vi "Field_C.vi"(8 "Queue to master":T10, 11 "Module queue":T10) -> ()   [LabVIEW 2024, in "Magnet module.lvlib"]
doc: "Magnet module controls: power supply unit (PSU/SMS) and temperature monitor (TM/LSC218).\nPSU controls mainly: switch heater and ramping of current which runs throught coil.\nTM controls temperature of switch, coil and cryostat.\nMessage for magnet is a cluster that contains: {(enum) Command , (variant) Data}\nFor simplifieing of documentation, the Command is noted as a name of instruction, and Data is represented by a requered datatype (mostly cluster) name.\nCommands:\nInitialize(Magnet Config Constants) - Sugesstion: Load configuration constants from configuration file.\nSet field (Set field{B, R, cr}) - B-field[T], R-ramp[A/s], cr - custom ramp[bool].\nSwitch mode(mode) - to persistant, or to ramping.\nBlackout() - undone functionality of emergency deenergizing.\nUpdate() - Important! This triggers update of data from instruments. Shoud occure in regular intervals as priority message.\nResponses:\nMagnet initialized ();\nTM revision(temperature monitor revision);\nMagnet init error(error);\nSetting field(Set Field{B, R, cr});\nWarning(string);\nSwitching to(mode);\nUpdate error(error);\nTM update(TM sensors);\nPSU update(PSU data);\nMagnet status();"
uses:
  Magnet module.lvlib
  ctl/SetField data.ctl
  ctl/RampingOutput.ctl
  ctl/Magnet mode.ctl
  ctl/Overall status.ctl
  ctl/Magnet config constants.ctl
  ctl/Cryostat temperature sensors.ctl
  Messenger service/Data types/Module name.ctl
  <instrlib>/SMS drivers/Public/PSU Status.ctl
  <instrlib>/SMS drivers/Cryogenic Ltd SMSXXX.lvlib
  ctl/Magnet Orders.ctl
  ctl/MSG to magnet.ctl
  ctl/Magnet mode public.ctl
  ctl/Actual magnet state.ctl
  Messenger service/Data types/Mailbox address.ctl
  Messenger service/MessengerLib.lvlib
panel:
  out "Time stamp":dbl format="%<%H:%M:%S%3u\n%Y/%m/%d>T"
  out "Connected":bool
  out "Magnet Constants":T1={"Switch resistant [K]"=5.0, "Switch superconducting [K]"=4.0, "First stage critical temperature [K]"=50.0, "Second stage critical temperature [K]"=5.0, "Inner magnet critical temperature [K]"=6.0, "Outer magnet critical temperature [K]"=5.0, "Field Constant [T/A]"=0.14911, "Maximum Current [A]"=107.3, "Maximum field [T]"=16.0, "Maximum source ramp [A/s]"=0.5, "Source precision [T]"=2e-05, "Ramp limits [A/s]"=[0.0506, 0.038, 0.0285, 0.0213, 0.0104], "Field limits [T]"=[3.0, 9.6, 13.3, 15.5, 16.0], "SMS"="", "LSC218"=""}
  out "Overall status":T2={"Desired"={"Field [T]"=0.0, "Ramp [T/s]"=0.0, "Custom Ramp?"=TRUE, "Mode"=enum."Persistant"}, "Actual"={"Mode"=enum."Persistant", "Ramping output"=enum."At Target", "Ready for change"=FALSE, "Switch heater"=FALSE, "Cooler Overheat"=FALSE, "Coil overheat"=FALSE, "Energized"=FALSE, "Output [T]"=0.0, "Field [T]"=0.0, "Ramp[T/s]"=0.0, "Switch\ntemperature [K]"=1.0, "Voltage [V]"=0.0, "Current direction"=FALSE}}
  out "Temperatures":T8 {"Time stamp" format="%<%H:%M:%S%2u\n%Y/%m/%d>T"}
  out "PSU Status Out":T9 {"Trip Current" format="%.3f"; "Trip Field" format="%.4f"; "Voltage" format="%.2f"; "Field Constant" format="%.6f"; "MID Setpoint (T)" format="%.4f"; "MID Setpoint (A)" format="%.3f"; "MAX Setpoint (T)" format="%.4f"; "MAX Setpoint (A)" format="%.3f"; "Heater Voltage" format="%.2f"; "V Limit (V)" format="%.2f"; "Ramp Rate (A/s)" format="%.3f"; "Output (A)" format="%.3f"; "Output (T)" format="%.4f"; "Persistent Current" format="%.3f"; "Persistent Field" format="%.4f"}
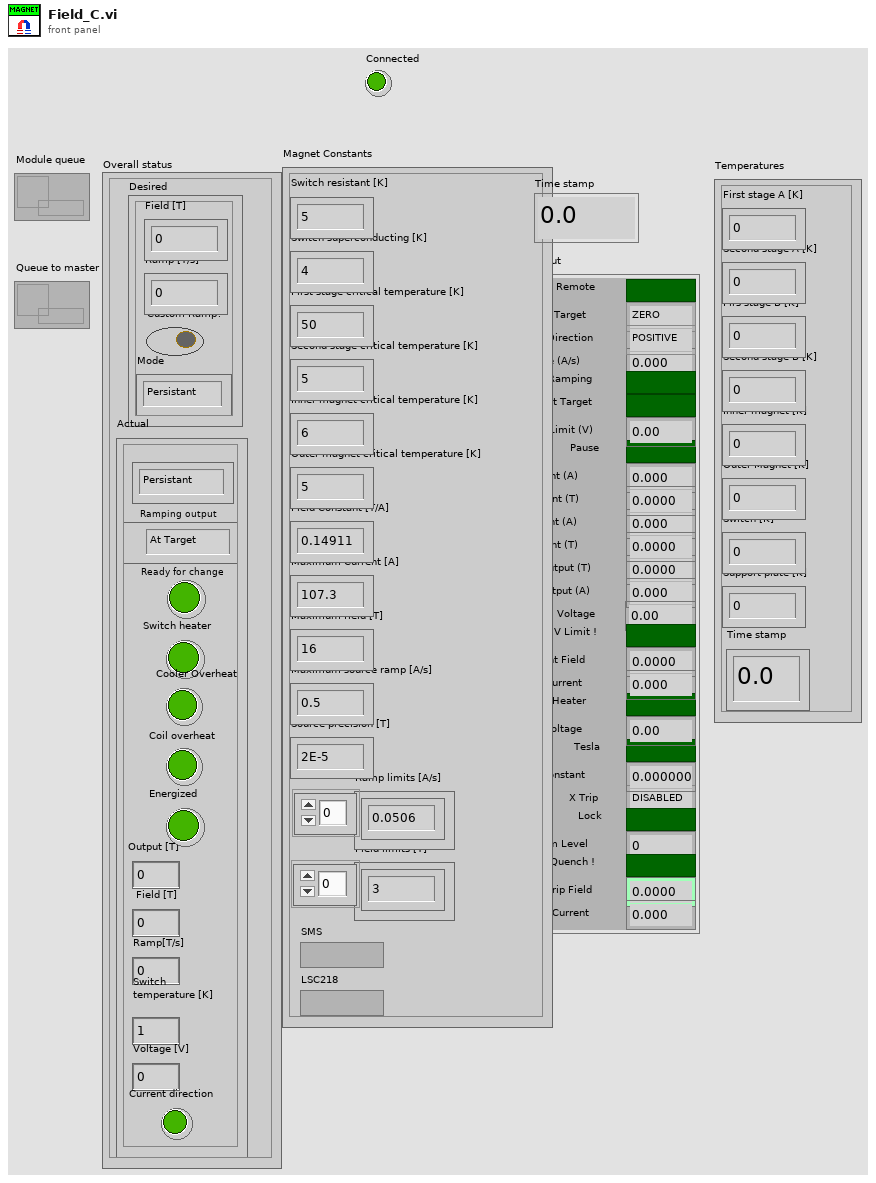
[diagram p1: front panel]
types:
  T1 = typedef "Magnet module.lvlib/Magnet config constants.ctl" = cluster{"Switch resistant [K]":dbl, "Switch superconducting [K]":dbl, "First stage critical temperature [K]":dbl, "Second stage critical temperature [K]":dbl, "Inner magnet critical temperature [K]":dbl, "Outer magnet critical temperature [K]":dbl, "Field Constant [T/A]":dbl, "Maximum Current [A]":dbl, "Maximum field [T]":dbl, "Maximum source ramp [A/s]":dbl, "Source precision [T]":dbl, "Ramp limits [A/s]":dbl[], "Field limits [T]":dbl[], "SMS":refnum<visa-resource-name>, "LSC218":refnum<visa-resource-name>}
  T2 = typedef "Magnet module.lvlib/Overall status.ctl" = cluster{"Desired":T3, "Actual":T5}
  T3 = typedef "Magnet module.lvlib/SetField data.ctl" = cluster{"Field [T]":dbl, "Ramp [T/s]":dbl, "Custom Ramp?":bool, "Mode":T4}
  T4 = typedef "Magnet module.lvlib/Magnet mode public.ctl" = enum16{"Persistant", "Ramping"}
  T5 = typedef "Magnet module.lvlib/Actual magnet state.ctl" = cluster{"Mode":T6, "Ramping output":T7, "Ready for change":bool, "Switch heater":bool, "Cooler Overheat":bool, "Coil overheat":bool, "Energized":bool, "Output [T]":dbl, "Field [T]":dbl, "Ramp[T/s]":dbl, "Switch\ntemperature [K]":dbl, "Voltage [V]":dbl, "Current direction":bool}
  T6 = typedef "Magnet module.lvlib/Magnet mode.ctl" = enum16{"Persistant", "Switching", "Ramping", "Quenched"}
  T7 = typedef "Magnet module.lvlib/RampingOutput.ctl" = enum16{"At Target", "Go up", "Go down"}
  T8 = typedef "Magnet module.lvlib/Cryostat temperature sensors.ctl" = cluster{"First stage A [K]":dbl, "Second stage A [K]":dbl, "Firs stage B [K]":dbl, "Second stage B [K]":dbl, "Inner magnet [K]":dbl, "Outer Magnet [K]":dbl, "Switch [K]":dbl, "Support plate [K]":dbl, "Time stamp":dbl}
  T9 = typedef "Cryogenic Ltd SMSXXX.lvlib/PSU Status.ctl" = cluster{"Ramp Target":enum16{"ZERO", "MID", "MAX"}, "Pause":bool, "Switch Heater":bool, "Persistent Field":dbl, "Persistent Current":dbl, "Tesla":bool, "Output (T)":dbl, "Output (A)":dbl, "X Trip":enum16{"DISABLED", "ENABLED", "ACTIVE"}, "Ramp Rate (A/s)":dbl, "V Limit (V)":dbl, "Heater Voltage":dbl, "MAX Setpoint (A)":dbl, "MAX Setpoint (T)":dbl, "MID Setpoint (A)":dbl, "MID Setpoint (T)":dbl, "Lock":bool, "Field Constant":dbl, "Remote":bool, "Direction":enum16{"POSITIVE", "NEGATIVE", "OPEN", "UNIPOLAR"}, "Helium Level":u16, "Quench !":bool, "Voltage":dbl, "V Limit !":bool, "Ramping":bool, "At Target":bool, "Trip Field":dbl, "Trip Current":dbl}
  T10 = typedef "MessengerLib.lvlib/Mailbox address.ctl" = refnum<queue>
  T11 = enum16{"Begin", "Idle", "Connect", "UpdateAll", "UpdateQuick", "Set field", "Set mode", "Emergency", "Disconnect", "Exit"}
  T12 = typedef "Module name.ctl" = enum16{"Emty", "Magnet", "VTI", "Excitation", "Servo", "Acquisition", "Rotator", "Digitizer", "SMU2450", "Carousel", "Multimeter", "Tmp monitor", "Power monitor"}
  T13 = typedef "Magnet module.lvlib/Magnet Orders.ctl" = enum16{"Ignore", "Connect", "Update", "Switch mode", "Set field", "Stop ramping", "Equalize output", "Zero output", "Flip polarity", "Blackout", "Set timer", "Eval temperatures", "Disconnect"}
  T14 = typedef "Magnet module.lvlib/MSG to magnet.ctl" = cluster{"Order":T13, "Data":variant}
  T15 = enum16{"POSITIVE", "NEGATIVE", "OPEN", "UNIPOLAR"}
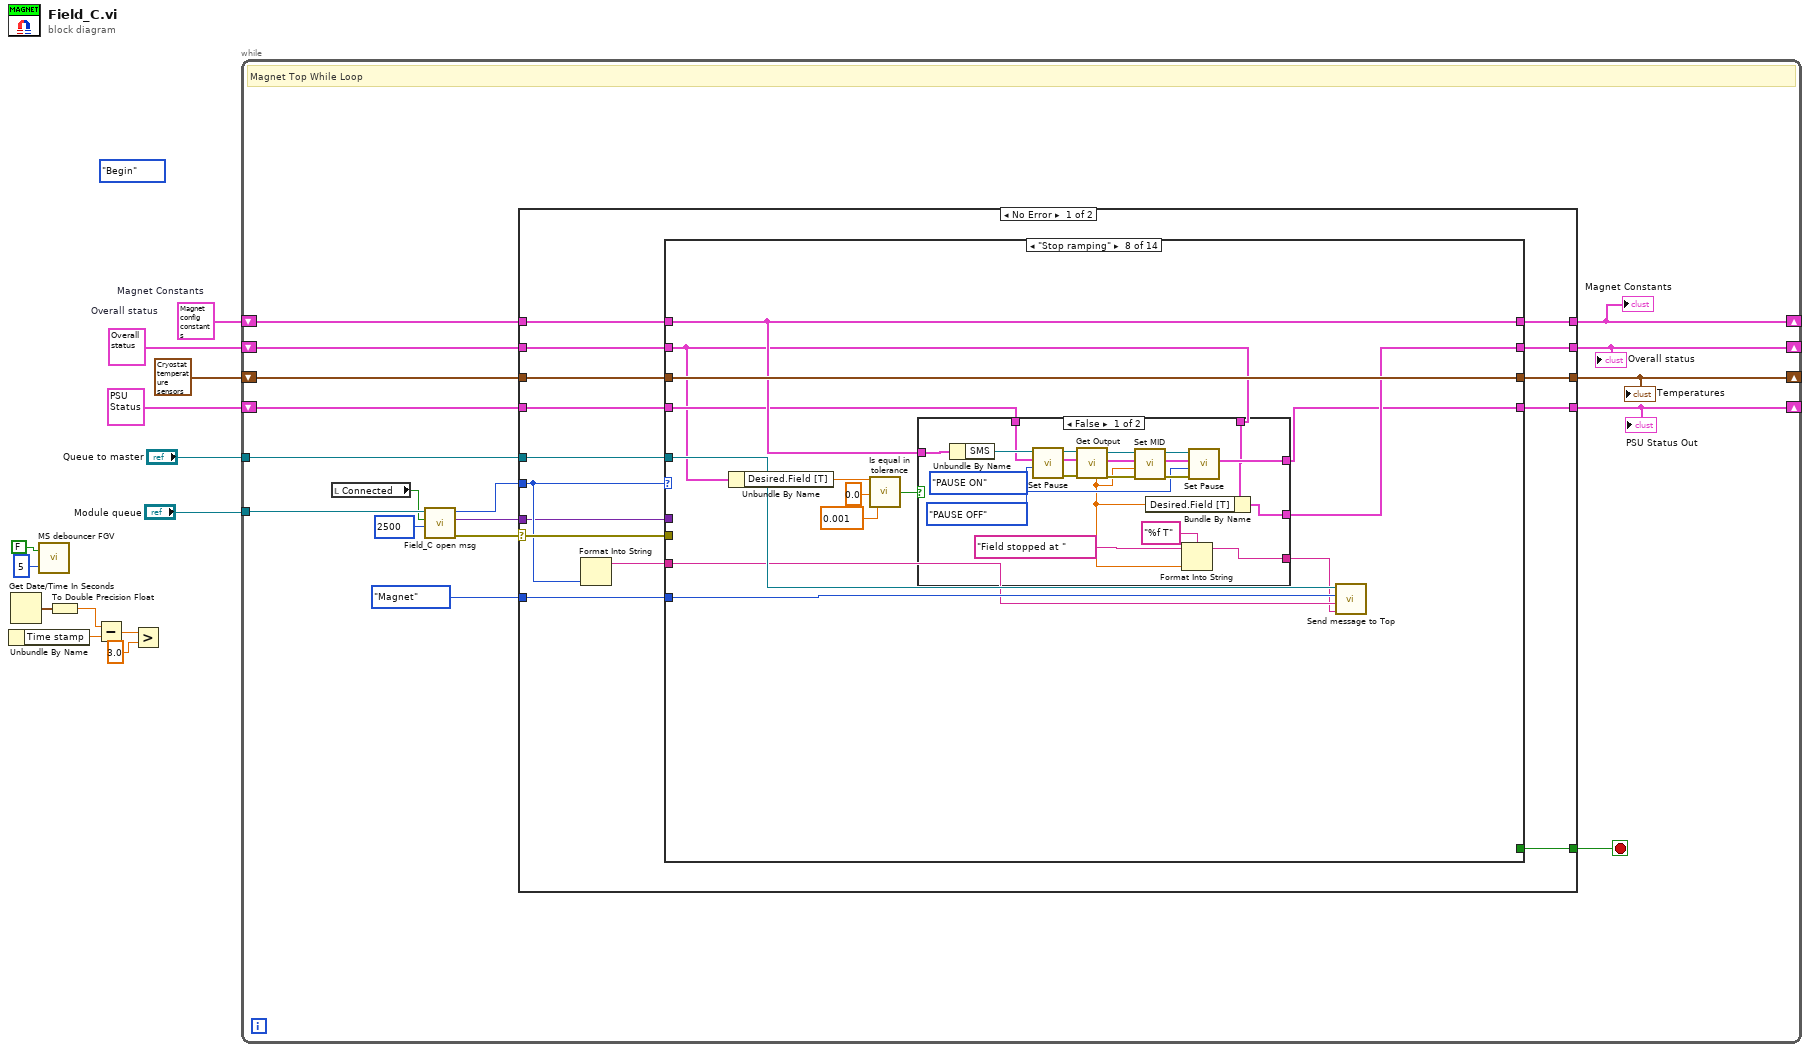
[diagram p0: block diagram]
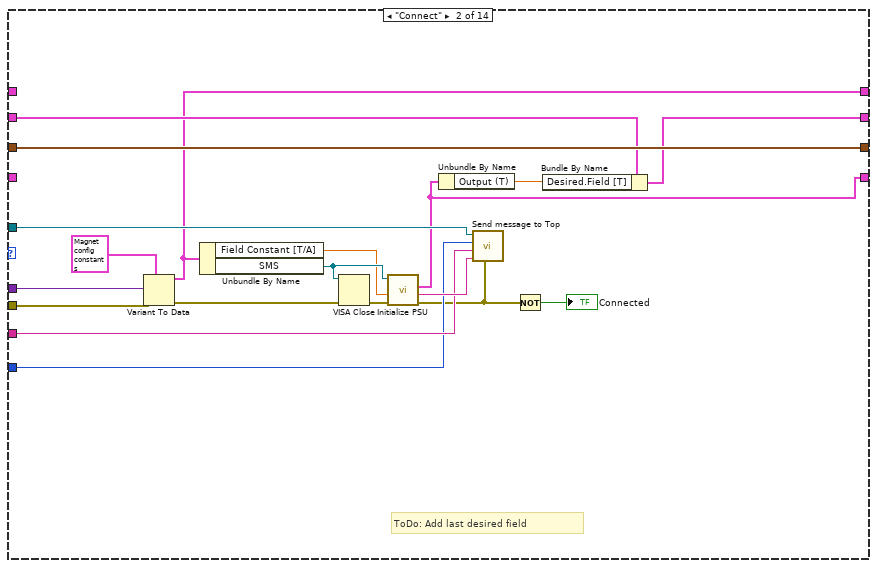
[diagram p3: hidden frame]
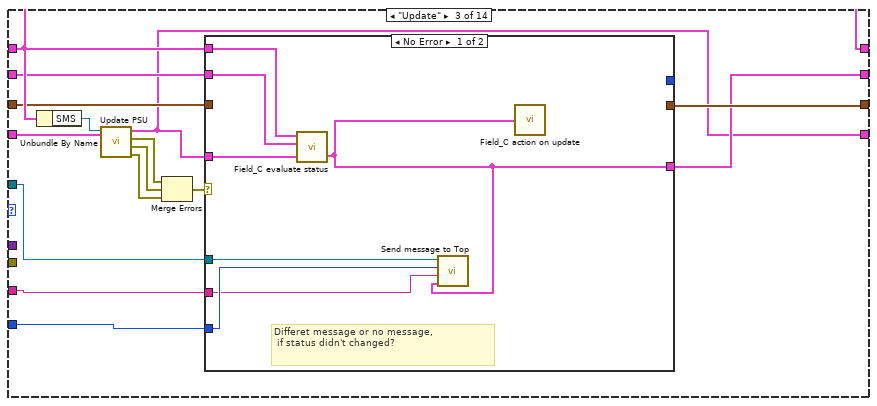
[diagram p4: hidden frame]
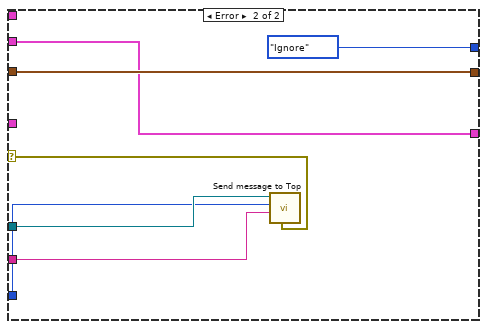
[diagram p5: hidden frame]
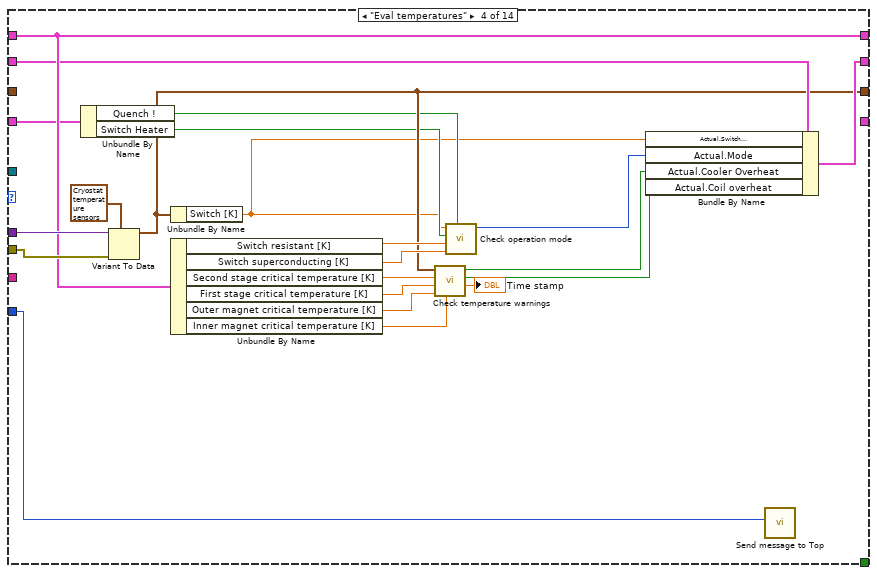
[diagram p6: hidden frame]
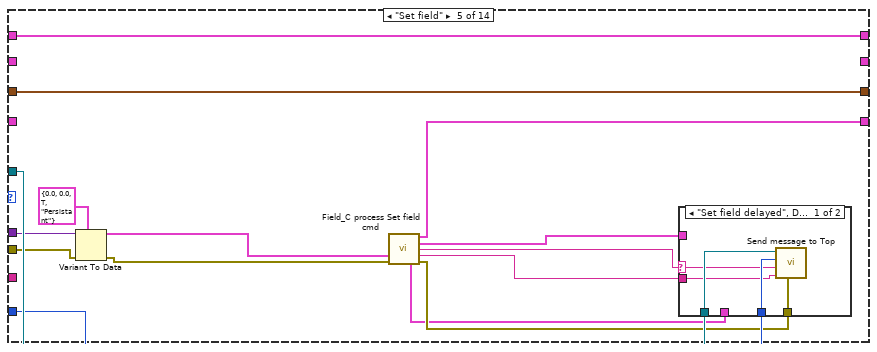
[diagram p7: hidden frame]
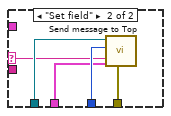
[diagram p8: hidden frame]
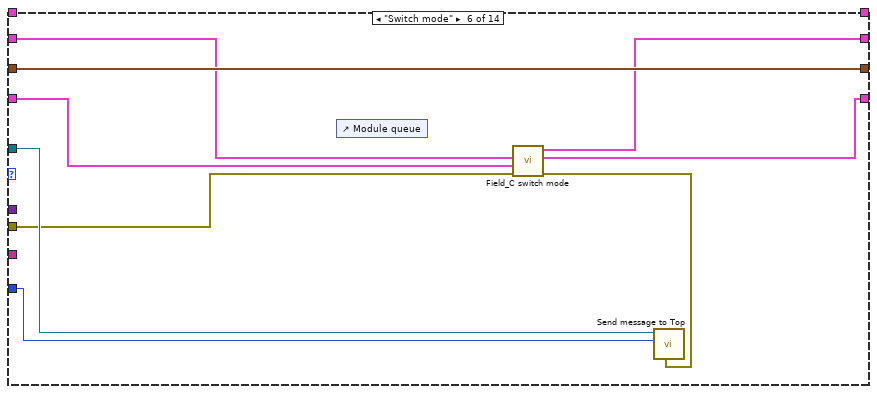
[diagram p9: hidden frame]
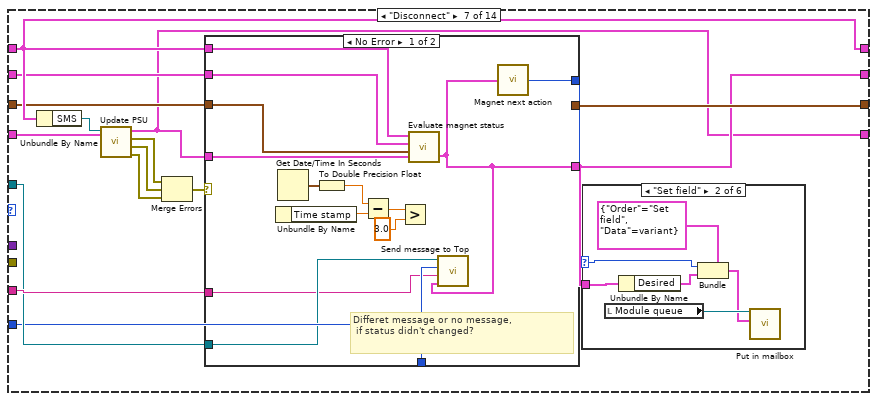
[diagram p10: hidden frame]
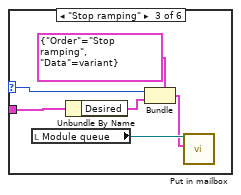
[diagram p12: hidden frame]
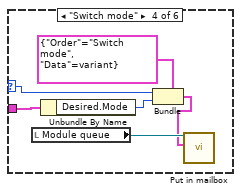
[diagram p13: hidden frame]
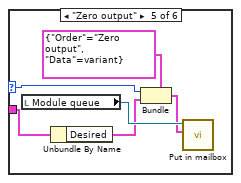
[diagram p14: hidden frame]
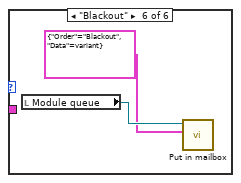
[diagram p15: hidden frame]
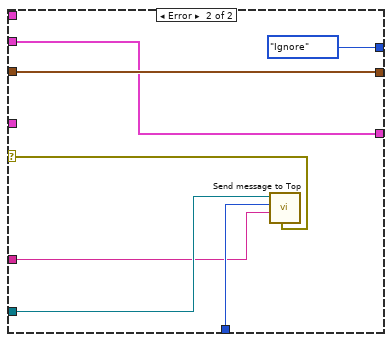
[diagram p16: hidden frame]
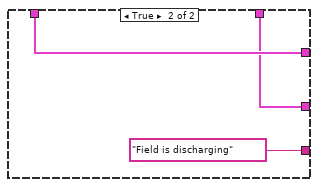
[diagram p17: hidden frame]
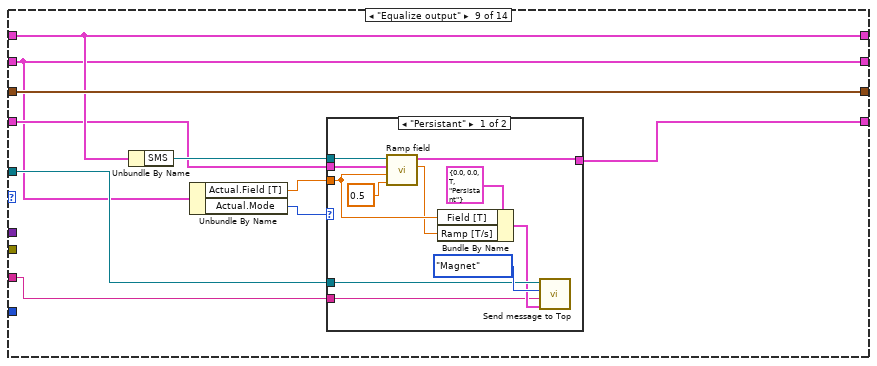
[diagram p18: hidden frame]
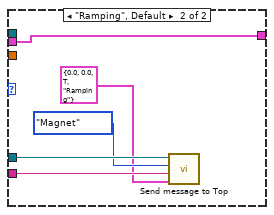
[diagram p19: hidden frame]
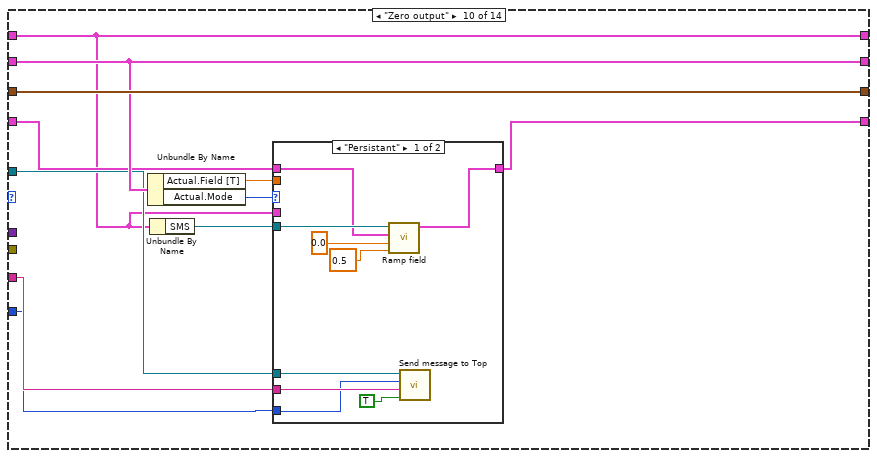
[diagram p20: hidden frame]
diagram:
  (unwired) T11."Begin"
  w6 = T1 {"Switch resistant [K]"=5.0, "Switch superconducting [K]"=4.0, "First stage critical temperature [K]"=50.0, "Second stage critical temperature [K]"=5.0, "Inner magnet critical temperature [K]"=6.0, "Outer magnet critical temperature [K]"=5.0, "Field Constant [T/A]"=0.14911, "Maximum Current [A]"=107.3, "Maximum field [T]"=16.0, "Maximum source ramp [A/s]"=0.5, "Source precision [T]"=2e-05, "Ramp limits [A/s]"=[0.0506, 0.038, 0.0285, 0.0213, 0.0104], "Field limits [T]"=[3.0, 9.6, 13.3, 15.5, 16.0], "SMS"="COM3", "LSC218"="COM1"}  # Magnet Constants
  w13 = T2 {"Desired"={"Field [T]"=0.0, "Ramp [T/s]"=0.0, "Custom Ramp?"=TRUE, "Mode"=enum."Persistant"}, "Actual"={"Mode"=enum."Persistant", "Ramping output"=enum."At Target", "Ready for change"=FALSE, "Switch heater"=FALSE, "Cooler Overheat"=FALSE, "Coil overheat"=FALSE, "Energized"=FALSE, "Output [T]"=0.0, "Field [T]"=0.0, "Ramp[T/s]"=0.0, "Switch\ntemperature [K]"=1.0, "Voltage [V]"=0.0, "Current direction"=FALSE}}  # Overall status
  n1 = Unbundle By Name() -> ("Time stamp"=w3:dbl)  [unwired: 1 in]
  n2 = Get Date/Time In Seconds() -> (seconds since 1Jan1904=w2:timestamp)
  n3 = call "MS debouncer FGV.vi"("Iterations"=5, "At target?"=FALSE ("On target?")) -> ()  [unwired: 1 out]
  n4 = To Double Precision Float(number=w2) -> (double precision float=w4:dbl)
  n5 = Subtract(x=w4, y=w3) -> (x-y=w5:dbl)
  n6 = Greater?(x=w5, y=3.0) -> ()  [unwired: 1 out]
  n7 = while {
    tunnel: "Module queue" -> [w30]
    tunnel: "Queue to master" -> [w29]
    shift-right: [w24] -> _
    shift-left: w13 -> [w25]
    shift-right: [w26] -> _
    shift-left: T8 {"First stage A [K]"=0.0, "Second stage A [K]"=0.0, "Firs stage B [K]"=0.0, "Second stage B [K]"=0.0, "Inner magnet [K]"=0.0, "Outer Magnet [K]"=0.0, "Switch [K]"=0.0, "Support plate [K]"=0.0, "Time stamp"=0.0} ("Temperatures") -> [w27]
    shift-right: [w23] -> _
    shift-left: T9 {"Ramp Target"=enum."ZERO", "Pause"=FALSE, "Switch Heater"=FALSE, "Persistent Field"=0.0, "Persistent Current"=0.0, "Tesla"=FALSE, "Output (T)"=0.0, "Output (A)"=0.0, "X Trip"=enum."DISABLED", "Ramp Rate (A/s)"=0.0, "V Limit (V)"=0.0, "Heater Voltage"=0.0, "MAX Setpoint (A)"=0.0, "MAX Setpoint (T)"=0.0, "MID Setpoint (A)"=0.0, "MID Setpoint (T)"=0.0, "Lock"=FALSE, "Field Constant"=0.0, "Remote"=FALSE, "Direction"=enum."POSITIVE", "Helium Level"=0, "Quench !"=FALSE, "Voltage"=0.0, "V Limit !"=FALSE, "Ramping"=FALSE, "At Target"=FALSE, "Trip Field"=0.0, "Trip Current"=0.0} ("PSU Status Out") -> [w22]
    shift-right: [w28] -> _
    shift-left: w6 -> [w21]
    stop <- w20 stop-if-true
    # "Magnet Top While Loop"
    n8 = local read "Connected"() -> (w16:bool)
    n9 = call "Field_C open msg.vi"("timeout ms (2500)"=2500 ("timeout in ms (-1)"), "Connected"=w16, "Queue in"=w30) -> ("error out 2"=w17:errorcluster, "Data"=w18:variant, "Command"=w15:T13)  [unwired: 4 in, 2 out]
    n10 = case shown="No Error" w17 {
      selector: w17 -> [w36 _]
      tunnel: w29 -> [w45 _]
      tunnel: w18 -> [w32 _]
      tunnel: [w44 w410] -> w24
      tunnel: w25 -> [w43 w410]
      tunnel: w21 -> [w42 w411]
      tunnel: [w41 w411] -> w28
      tunnel: w27 -> [w40 w409]
      tunnel: [w39 w409] -> w26
      tunnel: [w38 w408] -> w23
      tunnel: w22 -> [w37 w408]
      tunnel: [w34 _] -> w20
      tunnel: w15 -> [w33 _]
      tunnel: Module_name."Magnet" ("Module") -> [w31 _]
      frame No Error {
        n11 = Format Into String(w33) -> (resulting string=w35:string)  [unwired: 3 in, 1 out]
        n12 = case shown="\"Stop ramping\"" w33 {
          tunnel: w45 -> [_ w68 w74 _ w132 w153 w160 w229 w259 w288 w319 _ w387 w396]
          tunnel: [w49 w64 w76 w118 _ w146 w162 w226 w258 w290 w323 w368 w389 w398] -> w44
          tunnel: w43 -> [w49 w65 w80 w107 _ w151 w166 w222 w258 w290 w323 w368 w389 w398]
          tunnel: w42 -> [w48 _ w81 w108 w123 _ w167 w225 w263 w282 w315 w371 w388 w397]
          tunnel: [w48 w58 w81 w108 w123 _ w167 w225 w263 w282 w315 w371 w388 w397] -> w41
          tunnel: w40 -> [w47 w67 w78 _ w134 w152 w164 w230 w264 w291 w324 w370 w393 w407]
          tunnel: [w47 w67 w77 w102 w134 w152 w163 w230 w264 w291 w324 w370 w393 w407] -> w39
          tunnel: [w46 w63 w72 _ w131 w149 w157 w223 w260 w285 w314 w369 w392 w406] -> w38
          tunnel: w37 -> [w46 _ w79 w106 _ w150 w165 w224 w261 w286 w316 w369 w392 w406]
          tunnel: w36 -> [_ w60 _ w109 w120 w145 _ _ _ _ w318 _ w383 _]
          tunnel: w31 -> [_ w56 w73 w119 w129 w148 w159 w228 _ w283 w321 _ w384 _]
          tunnel: w35 -> [_ w57 w75 _ _ _ w161 w227 w255 w284 w320 _ w386 w394]
          tunnel: [_ _ _ _ _ _ _ _ _ _ _ _ w380 FALSE] -> w34
          tunnel: w32 -> [_ w52 _ w111 w121 _ _ _ _ _ _ _ w382 _]
          frame "Ignore", Default {
          }
          frame "Connect" {
            # "ToDo: Add last desired field"
            n13 = Variant To Data(error in=w60, type=T1 {"Switch resistant [K]"=5.0, "Switch superconducting [K]"=4.0, "First stage critical temperature [K]"=50.0, "Second stage critical temperature [K]"=5.0, "Inner magnet critical temperature [K]"=6.0, "Outer magnet critical temperature [K]"=5.0, "Field Constant [T/A]"=0.14911, "Maximum Current [A]"=107.3, "Maximum field [T]"=16.0, "Maximum source ramp [A/s]"=0.5, "Source precision [T]"=2e-05, "Ramp limits [A/s]"=[0.0506, 0.038, 0.0285, 0.0213, 0.0104], "Field limits [T]"=[3.0, 9.6, 13.3, 15.5, 16.0], "SMS"="", "LSC218"=""} ("Magnet Config Constants"), Variant=w52) -> (data=w58:T1, error out=w59:errorcluster)
            n14 = Unbundle By Name(w58) -> ("Field Constant [T/A]"=w53:dbl, "SMS"=w55:refnum<visa-resource-name>)
            n15 = VISA Close(VISA resource name=w55, error in (no error)=w59) -> (error out=w54:errorcluster)
            n16 = call "Initialize PSU.vi"("error in"=w54, "Field Constant"=w53, "PSU VISA name"=w55) -> ("error out"=w50:errorcluster, "Initial message"=w66:string, "initial PSU Status"=w63:T9)  [unwired: 6 in]
            n17 = Unbundle By Name(w63) -> ("Output (T)"=w62:dbl)
            n18 = call "Send message to Top.vi"("Error in (no error)"=w50, "Data"=w66, "Response"=w57, "Module"=w56, "Mailbox address in"=w68) -> ()  [unwired: 5 in, 2 out]
            n19 = Not(x=w50) -> (.not. x?=→"Connected":bool)
            n20 = Bundle By Name(cluster=w65, "Desired.Field [T]"=w62) -> (w64:T2)
          }
          frame "Update" {
            n21 = Unbundle By Name(w81) -> ("SMS"=w83:refnum<visa-resource-name>)
            n22 = call "Update PSU.vi"("PSU Status In"=w79, "VISA Resource Name In"=w83) -> ("Output err"=w82:errorcluster, "Ramp state err"=w69:errorcluster, "Sign err"=w70:errorcluster, "PSU Status Out"=w72:T9)  [unwired: 2 in]
            n23 = Merge Errors(w70, w69, w82) -> (w71:errorcluster)
            n24 = case shown="No Error" w71 {
              selector: w71 -> [_ w93]
              tunnel: w74 -> [w90 w96]
              tunnel: w72 -> [w89 _]
              tunnel: [w84 w95] -> w76
              tunnel: w78 -> [_ w97]
              tunnel: [_ w97] -> w77
              tunnel: w81 -> [w88 _]
              tunnel: w80 -> [w87 w95]
              tunnel: w73 -> [w86 w94]
              tunnel: w75 -> [w85 w92]
              tunnel: [_ Magnet_Orders."Ignore" ("Command out")] -> _
              frame No Error {
                # "Differet message or no message,\n if status didn't changed?"
                n25 = call "Field_C evaluate status.vi"("PSU Status in"=w89, "Overall status in"=w87, "Magnet Constants"=w88) -> ("Overall status out"=w84:T2)  [unwired: 2 in]
                n26 = call "Send message to Top.vi"("Data"=w84, "Response"=w85, "Module"=w86, "Mailbox address in"=w90) -> ()  [unwired: 6 in, 2 out]
                n27 = call "Field_C action on update.vi"("Overall status in"=w84) -> ()  [unwired: 3 in, 2 out]
              }
              frame Error {
                n28 = call "Send message to Top.vi"("Error in (no error)"=w93, "Response"=w92, "Module"=w94, "Mailbox address in"=w96) -> ()  [unwired: 6 in, 2 out]
              }
            }
          }
          frame "Eval temperatures" {
            n29 = Unbundle By Name(w106) -> ("Quench !"=w99:bool, "Switch Heater"=w100:bool)
            n30 = Variant To Data(error in=w109, type=T8 {"First stage A [K]"=0.0, "Second stage A [K]"=0.0, "Firs stage B [K]"=0.0, "Second stage B [K]"=0.0, "Inner magnet [K]"=0.0, "Outer Magnet [K]"=0.0, "Switch [K]"=0.0, "Support plate [K]"=0.0, "Time stamp"=0.0} ("Temperatures"), Variant=w111) -> (data=w102:T8)  [unwired: 1 out]
            n31 = Unbundle By Name(w102) -> ("Switch [K]"=w98:dbl)
            n32 = Unbundle By Name(w108) -> ("Switch resistant [K]"=w113:dbl, "Switch superconducting [K]"=w112:dbl, "Second stage critical temperature [K]"=w114:dbl, "First stage critical temperature [K]"=w115:dbl, "Outer magnet critical temperature [K]"=w116:dbl, "Inner magnet critical temperature [K]"=w117:dbl)
            n33 = call "Check temperature warnings.vi"("Inner coil limit [K]"=w117, "Outer coil limit [K]"=w116, "1st Cryocooler limit [K]"=w115, "2nd cryocooler limit [K]"=w114, "LSC218 sensors"=w102) -> ("Time stamp"=→"Time stamp":dbl, "Coil Overheat"=w104:bool, "Crocooler overheat"=w105:bool)  [unwired: 4 in]
            n34 = call "Check operation mode.vi"("Quenched?"=w99, "Switch supercond [K]"=w112, "Switch rezist [K]"=w113, "Switch Heater"=w100, "Switch actual [K]"=w98) -> ("Magnet Mode"=w103:T6)  [unwired: 6 in]
            n35 = Bundle By Name(cluster=w107, "Actual.Switch\ntemperature [K]"=w98, "Actual.Mode"=w103, "Actual.Cooler Overheat"=w105, "Actual.Coil overheat"=w104) -> (w118:T2)
            n36 = call "Send message to Top.vi"("Module"=w119) -> ()  [unwired: 9 in, 2 out]
          }
          frame "Set field" {
            n37 = Variant To Data(error in=w120, type=T3 {"Field [T]"=0.0, "Ramp [T/s]"=0.0, "Custom Ramp?"=TRUE, "Mode"=enum."Persistant"} ("Set Field"), Variant=w121) -> (data=w130:T3, error out=w128:errorcluster)
            n38 = call "Field_C process Set field cmd.vi"(9:w130, "error in (no error)"=w128) -> ("PSU Status Out out"=w131:T9, "Overall status out"=w127:T2, "Cmd response"=w126:string, "String out"=w122:string, "Desired"=w124:T3, "error out"=w125:errorcluster)  [unwired: 8 in]
            n39 = case shown="\"Set field delayed\", Default" w126 {
              selector: w126 -> [w137 w141]
              tunnel: w132 -> [w139 w144]
              tunnel: w129 -> [w138 w143]
              tunnel: w125 -> [w136 w142]
              tunnel: w127 -> [_ _]
              tunnel: w124 -> [_ w140]
              tunnel: w122 -> [w135 _]
              frame "Set field delayed", Default {
                n40 = call "Send message to Top.vi"("Error in (no error)"=w136, "Data"=w135, "Response"=w137, "Module"=w138, "Mailbox address in"=w139) -> ()  [unwired: 5 in, 2 out]
              }
              frame "Set field" {
                n41 = call "Send message to Top.vi"("Error in (no error)"=w142, "Data"=w140, "Response"=w141, "Module"=w143, "Mailbox address in"=w144) -> ()  [unwired: 5 in, 2 out]
              }
            }
          }
          frame "Switch mode" {
            n42 = control-ref of="Module queue"() -> ()  [unwired: 1 out]
            n43 = call "Field_C switch mode.vi"("error in (no error)"=w145, "PSU Status"=w150, "Overall status in"=w151) -> ("error out"=w147:errorcluster, "PSU Status out"=w149:T9, "Overall status out"=w146:T2)  [unwired: 6 in]
            n44 = call "Send message to Top.vi"("Error in (no error)"=w147, "Module"=w148, "Mailbox address in"=w153) -> ()  [unwired: 7 in, 2 out]
          }
          frame "Disconnect" {
            n45 = Unbundle By Name(w167) -> ("SMS"=w169:refnum<visa-resource-name>)
            n46 = call "Update PSU.vi"("PSU Status In"=w165, "VISA Resource Name In"=w169) -> ("Output err"=w168:errorcluster, "Ramp state err"=w154:errorcluster, "Sign err"=w155:errorcluster, "PSU Status Out"=w157:T9)  [unwired: 2 in]
            n47 = Merge Errors(w155, w154, w168) -> (w156:errorcluster)
            n48 = case shown="No Error" w156 {
              selector: w156 -> [_ w212]
              tunnel: w160 -> [w209 w215]
              tunnel: w157 -> [w208 _]
              tunnel: [w202 w214] -> w162
              tunnel: w164 -> [w196 w216]
              tunnel: [_ w216] -> w163
              tunnel: w167 -> [w207 _]
              tunnel: w166 -> [w206 w214]
              tunnel: w159 -> [w205 w213]
              tunnel: w161 -> [w204 w211]
              tunnel: [w203 Magnet_Orders."Ignore" ("Command out")] -> w158
              frame No Error {
                # "Differet message or no message,\n if status didn't changed?"
                n49 = Unbundle By Name() -> ("Time stamp"=w200:dbl)  [unwired: 1 in]
                n50 = Get Date/Time In Seconds() -> (seconds since 1Jan1904=w201:timestamp)
                n51 = To Double Precision Float(number=w201) -> (double precision float=w199:dbl)
                n52 = Subtract(x=w199, y=w200) -> (x-y=w198:dbl)
                n53 = Greater?(x=w198, y=3.0) -> ()  [unwired: 1 out]
                n54 = call "Evaluate magnet status.vi"("PSU Status in"=w208, "LSC218 sensors"=w196, "Overall status in"=w206, "Magnet Constants"=w207) -> ("Overall status out"=w202:T2)  [unwired: 1 in]
                n55 = call "Send message to Top.vi"("Data"=w202, "Response"=w204, "Module"=w205, "Mailbox address in"=w209) -> ()  [unwired: 6 in, 2 out]
                n56 = call "Magnet next action.vi"("Overall status in"=w202) -> ("Command out"=w203:T13)  [unwired: 3 in, 1 out]
              }
              frame Error {
                n57 = call "Send message to Top.vi"("Error in (no error)"=w212, "Response"=w211, "Module"=w213, "Mailbox address in"=w215) -> ()  [unwired: 6 in, 2 out]
              }
            }
            n58 = case shown="\"Set field\"" w158 {
              selector: w158 -> [_ w170 w176 w182 w188 _]
              tunnel: w162 -> [_ w172 w178 w184 w190 _]
              frame "Update", Default {
              }
              frame "Set field" {
                n59 = local read "Module queue"() -> (w175:T10)
                n60 = Unbundle By Name(w172) -> ("Desired"=w173:T3)
                n61 = Bundle(cluster=T14 {"Order"=enum."Set field", "Data"=variant} ("MSG to magnet"), "Order"=w170, "Data"=w173) -> (w171:T14)
                n62 = call "Put in mailbox.vi"("Message"=w171, "Queue in"=w175) -> ()  [unwired: 7 in, 3 out]
              }
              frame "Stop ramping" {
                n63 = local read "Module queue"() -> (w181:T10)
                n64 = Unbundle By Name(w178) -> ("Desired"=w179:T3)
                n65 = Bundle(cluster=T14 {"Order"=enum."Stop ramping", "Data"=variant} ("MSG to magnet"), "Order"=w176, "Data"=w179) -> (w177:T14)
                n66 = call "Put in mailbox.vi"("Message"=w177, "Queue in"=w181) -> ()  [unwired: 7 in, 3 out]
              }
              frame "Switch mode" {
                n67 = local read "Module queue"() -> (w187:T10)
                n68 = Unbundle By Name(w184) -> ("Desired.Mode"=w185:T4)
                n69 = Bundle(cluster=T14 {"Order"=enum."Switch mode", "Data"=variant} ("MSG to magnet"), "Order"=w182, "Data"=w185) -> (w183:T14)
                n70 = call "Put in mailbox.vi"("Message"=w183, "Queue in"=w187) -> ()  [unwired: 7 in, 3 out]
              }
              frame "Zero output" {
                n71 = local read "Module queue"() -> (w193:T10)
                n72 = Unbundle By Name(w190) -> ("Desired"=w191:T3)
                n73 = Bundle(cluster=T14 {"Order"=enum."Zero output", "Data"=variant} ("MSG to magnet"), "Order"=w188, "Data"=w191) -> (w189:T14)
                n74 = call "Put in mailbox.vi"("Message"=w189, "Queue in"=w193) -> ()  [unwired: 7 in, 3 out]
              }
              frame "Blackout" {
                n75 = local read "Module queue"() -> (w195:T10)
                n76 = call "Put in mailbox.vi"("Message"=T14 {"Order"=enum."Blackout", "Data"=variant} ("MSG to magnet"), "Queue in"=w195) -> ()  [unwired: 7 in, 3 out]
              }
            }
          }
          frame "Stop ramping" {
            n77 = Unbundle By Name(w222) -> ("Desired.Field [T]"=w221:dbl)
            n78 = call "Is equal in tolerance.vi"("Absolut tolerance"=0.001, "Reference value"=0.0, "Input value"=w221) -> ("Is in range"=w218:bool)  [unwired: 1 in]
            n79 = case shown="False" w218 {
              tunnel: [w251 w253] -> w226
              tunnel: w225 -> [w250 _]
              tunnel: w224 -> [w243 w254]
              tunnel: [w237 w254] -> w223
              tunnel: w222 -> [w235 w253]
              tunnel: [w233 "Field is discharging"] -> w217
              frame False {
                n80 = Unbundle By Name(w250) -> ("SMS"=w246:refnum<visa-resource-name>)
                n81 = call <instrlib>:"Set Pause.vi"("Pause (On/Off)"=enum16{"PAUSE OFF", "PAUSE ON"}."PAUSE ON", "PSU Status In"=w243, "VISA Resource Name IN"=w246) -> ("Error out"=w241:errorcluster, "PSU Status Out"=w242:T9, "VISA Resource Name Out"=w245:refnum<visa-resource-name>)  [unwired: 5 in, 1 out]
                n82 = call <instrlib>:"Get Output.vi"("Error in (no error)"=w241, "PSU Status In"=w242, "VISA Resource Name In"=w245) -> ("Error out"=w248:errorcluster, "PSU Status Out"=w249:T9, "VISA Resource Name Out"=w247:refnum<visa-resource-name>, "Output (T)"=w231:dbl)  [unwired: 3 in, 2 out]
                n83 = call <instrlib>:"Set MID.vi"("Error in (no error)"=w248, "MID (T or A)"=w231, "PSU Status In"=w249, "VISA Resource Name In"=w247) -> ("Error out"=w240:errorcluster, "PSU Status Out"=w238:T9, "VISA Resource Name Out"=w239:refnum<visa-resource-name>)  [unwired: 4 in, 1 out]
                n84 = Bundle By Name(cluster=w235, "Desired.Field [T]"=w231) -> (w251:T2)
                n85 = Format Into String(format string="%f T", initial string="Field stopped at ", w231) -> (resulting string=w233:string)  [unwired: 1 in, 1 out]
                n86 = call <instrlib>:"Set Pause.vi"("Error in (no error)"=w240, "Pause (On/Off)"=enum16{"PAUSE OFF", "PAUSE ON"}."PAUSE OFF", "PSU Status In"=w238, "VISA Resource Name IN"=w239) -> ("PSU Status Out"=w237:T9)  [unwired: 4 in, 3 out]
              }
              frame True {
              }
            }
            n87 = call "Send message to Top.vi"("Data"=w217, "Response"=w227, "Module"=w228, "Mailbox address in"=w229) -> ()  [unwired: 6 in, 2 out]
          }
          frame "Equalize output" {
            n88 = Unbundle By Name(w263) -> ("SMS"=w262:refnum<visa-resource-name>)
            n89 = Unbundle By Name(w258) -> ("Actual.Field [T]"=w256:dbl, "Actual.Mode"=w257:T6)
            n90 = case shown="\"Persistant\"" w257 {
              tunnel: w262 -> [w275 _]
              tunnel: w256 -> [w268 _]
              tunnel: w261 -> [w274 w280]
              tunnel: [w273 w280] -> w260
              tunnel: w259 -> [w271 w279]
              tunnel: w255 -> [w265 w277]
              frame "Persistant" {
                n91 = call "Ramp field.vi"("Ramp to set [A/s]"=0.5, "Field to set [T]"=w268, "PSU Status In"=w274, "VISA Refnum in"=w275) -> ("Ramp Rate (T/s)"=w266:dbl, "PSU Status Out"=w273:T9)  [unwired: 4 in, 2 out]
                n92 = Bundle By Name(cluster=T3 {"Field [T]"=0.0, "Ramp [T/s]"=0.0, "Custom Ramp?"=TRUE, "Mode"=enum."Persistant"} ("Desired"), "Field [T]"=w268, "Ramp [T/s]"=w266) -> (w267:T3)
                n93 = call "Send message to Top.vi"("Data"=w267, "Response"=w265, "Module"=Module_name."Magnet", "Mailbox address in"=w271) -> ()  [unwired: 6 in, 2 out]
              }
              frame "Ramping", Default {
                n94 = call "Send message to Top.vi"("Data"=T3 {"Field [T]"=0.0, "Ramp [T/s]"=0.0, "Custom Ramp?"=TRUE, "Mode"=enum."Ramping"} ("Desired"), "Response"=w277, "Module"=Module_name."Magnet", "Mailbox address in"=w279) -> ()  [unwired: 6 in, 2 out]
              }
            }
          }
          frame "Zero output" {
            n95 = Unbundle By Name(w290) -> ("Actual.Field [T]"=w281:dbl, "Actual.Mode"=w289:T6)
            n96 = Unbundle By Name(w282) -> ("SMS"=w287:refnum<visa-resource-name>)
            n97 = case shown="\"Persistant\"" w289 {
              tunnel: w288 -> [w300 w312]
              tunnel: w287 -> [w299 w301]
              tunnel: w286 -> [w298 w306]
              tunnel: [w297 w305] -> w285
              tunnel: w284 -> [w294 w310]
              tunnel: w283 -> [w292 w309]
              tunnel: w282 -> [_ w303]
              tunnel: w281 -> [_ w302]
              frame "Persistant" {
                n98 = call "Ramp field.vi"("Ramp to set [A/s]"=0.5, "Field to set [T]"=0.0, "PSU Status In"=w298, "VISA Refnum in"=w299) -> ("PSU Status Out"=w297:T9)  [unwired: 4 in, 3 out]
                n99 = call "Send message to Top.vi"("Data"=TRUE, "Response"=w294, "Module"=w292, "Mailbox address in"=w300) -> ()  [unwired: 6 in, 2 out]
              }
              frame "Ramping", Default {
                n100 = call "Next ramp and field.vi"("Magnet Constants in"=w303, "Actual field [T]"=w302, "Desired"=T3 {"Field [T]"=0.0, "Ramp [T/s]"=0.0, "Custom Ramp?"=FALSE, "Mode"=enum."Ramping"}) -> ("Ramp to set [A/s]"=w307:dbl, "Field to set [T]"=w308:dbl)  [unwired: 1 in]
                n101 = call "Ramp field.vi"("Ramp to set [A/s]"=w307, "Field to set [T]"=w308, "PSU Status In"=w306, "VISA Refnum in"=w301) -> ("PSU Status Out"=w305:T9)  [unwired: 4 in, 3 out]
                n102 = call "Send message to Top.vi"("Data"=FALSE, "Response"=w310, "Module"=w309, "Mailbox address in"=w312) -> ()  [unwired: 6 in, 2 out]
              }
            }
          }
          frame "Flip polarity" {
            n103 = Unbundle By Name(w323) -> ("Actual.Mode"=w322:T6)
            n104 = Variant To Data(error in=w318, type=TRUE) -> (data=w313:bool)  [unwired: 1 in, 1 out]
            n105 = case shown="\"Ramping\"" w322 {
              tunnel: w321 -> [w328 w342]
              tunnel: w320 -> [w327 w341]
              tunnel: w319 -> [w326 w340]
              tunnel: w316 -> [w329 w336]
              tunnel: [w329 w339] -> w314
              tunnel: w315 -> [_ w338]
              tunnel: w313 -> [_ w335]
              frame "Persistant", Default {
                n106 = call "Send message to Top.vi"("Data"="Cannot flip polarity", "Response"=w327, "Module"=w328, "Mailbox address in"=w326) -> ()  [unwired: 6 in, 2 out]
              }
              frame "Ramping" {
                n107 = Unbundle By Name(w336) -> ("Direction"=w330:T15)
                n108 = case shown="\"OPEN\"" w330 {
                  tunnel: w335 -> [w357 w360 _ _]
                  tunnel: [w356 w360 _ _] -> w334
                  tunnel: [enum16{"NEGATIVE", "POSITIVE"}."NEGATIVE" ("Current Direction") enum16{"NEGATIVE", "POSITIVE"}."POSITIVE" ("Current Direction") enum16{"NEGATIVE", "POSITIVE"}."POSITIVE" ("Current Direction") enum16{"NEGATIVE", "POSITIVE"}."POSITIVE" ("Current Direction")] -> w333
                  frame "POSITIVE", Default {
                    n109 = Not(x=w357) -> (.not. x?=w356:bool)
                  }
                  frame "NEGATIVE" {
                  }
                  frame "OPEN" {
                  }
                  frame "UNIPOLAR" {
                  }
                }
                n110 = Unbundle By Name(w338) -> ("SMS"=w337:refnum<visa-resource-name>)
                n111 = case shown="True" w334 {
                  tunnel: [w350 w353] -> w339
                  tunnel: w337 -> [w349 _]
                  tunnel: w336 -> [w348 w353]
                  tunnel: w333 -> [w346 _]
                  tunnel: [w345 w355] -> w332
                  tunnel: [w344 w354] -> w331
                  tunnel: w330 -> [_ w352]
                  frame True {
                    n112 = call <instrlib>:"Set Current Direction.vi"("Current Direction"=w346, "PSU Status In"=w348, "VISA Resource Name In"=w349) -> ("Error out"=w347:errorcluster, "PSU Status Out"=w350:T9)  [unwired: 5 in, 2 out]
                    n113 = Format Into String(format string="Set polarity: %s", error in=w347, w346) -> (resulting string=w345:string, error out=w344:errorcluster)  [unwired: 1 in]
                  }
                  frame False {
                    n114 = Format Into String(format string="Polarity is %s", w352) -> (resulting string=w355:string, error out=w354:errorcluster)  [unwired: 2 in]
                  }
                }
                n115 = call "Send message to Top.vi"("Error in (no error)"=w331, "Data"=w332, "Response"=w341, "Module"=w342, "Mailbox address in"=w340) -> ()  [unwired: 5 in, 2 out]
              }
            }
          }
          frame "Blackout" {
            n116 = Unbundle By Name(w368) -> ("Actual.Mode"=w366:T6, "Actual.Energized"=w367:bool, "Desired.Field [T]"=w363:dbl)
            n117 = Not Equal To 0?(x=w363) -> (x != 0?=w364:bool)
            n118 = And(x=w367, y=w364) -> (x .and. y?=w365:bool)
            n119 = case shown="True" w365 {
              tunnel: w366 -> [_ w372]
              frame False {
              }
              frame True {
                n120 = case shown="\"Persistant\", Default" w372 {
                  frame "Persistant", Default {
                    n121 = local read "Module queue"() -> (w378:T10)
                    n122 = Bundle(cluster=T14 {"Order"=enum."Set field", "Data"=variant} ("MSG to magnet"), "Order"=Magnet_Orders."Set field", "Data"=T3 {"Field [T]"=0.0, "Ramp [T/s]"=1.0, "Custom Ramp?"=FALSE, "Mode"=enum."Ramping"} ("Set Field")) -> (w377:T14)
                    n123 = call "Put in mailbox.vi"("Priority? (F)"=TRUE, "Message"=w377, "Queue in"=w378) -> ()  [unwired: 6 in, 3 out]
                  }
                  frame "Quenched" {
                  }
                }
              }
            }
          }
          frame "Disconnect" {
            n124 = Variant To Data(error in=w383, type=TRUE, Variant=w382) -> (data=w380:bool, error out=w379:errorcluster)
            n125 = Unbundle By Name(w388) -> ("SMS"=w391:refnum<visa-resource-name>)
            n126 = VISA Close(VISA resource name=w391, error in (no error)=w379) -> (error out=w390:errorcluster)
            n127 = call "Send message to Top.vi"("Data"=w390, "Response"=w386, "Module"=w384, "Mailbox address in"=w387) -> ()  [unwired: 6 in, 2 out]
            n128 = local write "Connected"(TRUE) -> ()
          }
          frame "Set timer" {
            n129 = Unbundle By Name(w397) -> ("LSC218"=w401:refnum<visa-resource-name>, "SMS"=w405:refnum<visa-resource-name>)
            n130 = VISA Close(VISA resource name=w405) -> (error out=w400:errorcluster)  [unwired: 1 in]
            n131 = VISA Close(VISA resource name=w401, error in (no error)=w400) -> (error out=w399:errorcluster)
            n132 = call "Send message to Top.vi"("Data"=w399, "Response"=w394, "Module"=Module_name."Magnet", "Mailbox address in"=w396) -> ()  [unwired: 6 in, 2 out]
            n133 = call "FGV magnet initialized.vi"("Write?(F)"=TRUE, "Initialized in"=FALSE) -> ()  [unwired: 9 in, 1 out]
          }
        }
      }
      frame Error {
      }
    }
    "PSU Status Out" <- w23
    "Temperatures" <- w26
    "Overall status" <- w24
    "Magnet Constants" <- w28
  }
